vi "Change Default Font.vi"(0 "PDF Report IN":refnum<class "PDF Report Class.lvclass">, 2 "Font":T1={"Name"="Helvetica", "Size"=12.0, "Color"=0, "Style"={"Bold"=FALSE, "Italic"=FALSE, "Underline"=FALSE, "Strikeout"=FALSE}, "Type"={"Type&direction"=enum."Select", "Embedded"=FALSE, "Encoding"=""}}, 11 "error in (no error)":errorcluster) -> (4 "PDF Report OUT":refnum<class "PDF Report Class.lvclass">, 15 "error out":errorcluster)   [LabVIEW 2019, in "Exaprom PDF.lvlib" / "Font Class.lvclass"]
doc: "Set the default font of the PDF report.\n\n<B>FRANÇAIS</B>\nChange la police de caractères par défaut du rapport PDF.\n\nDeveloped by Jean-Marc Simard\nCopyright © 2010, Exaprom Inc.\nAll rights reserved.\nLicense: BSD\n\nWith iTextSharp 4.1.6 (http://itextsharp.sourceforge.net)\nunder Mozilla Public License Version 1.1\n(http://www.mozilla.org/MPL/MPL-1.1.html)"
uses:
  Font Class.lvclass
  PDF Report Class/PDF Report Class.lvclass
  Controls/Font Controls/Font complete cluster.ctl
  Controls/Font Controls/Font size.ctl
  Controls/Font Controls/Font color.ctl
  Controls/Font Controls/Type and encoding.ctl
  Controls/Text Controls/Unicode/Type and run direction.ctl
  Font Class.lvclass/Font Class.ctl
  Exaprom PDF.lvlib
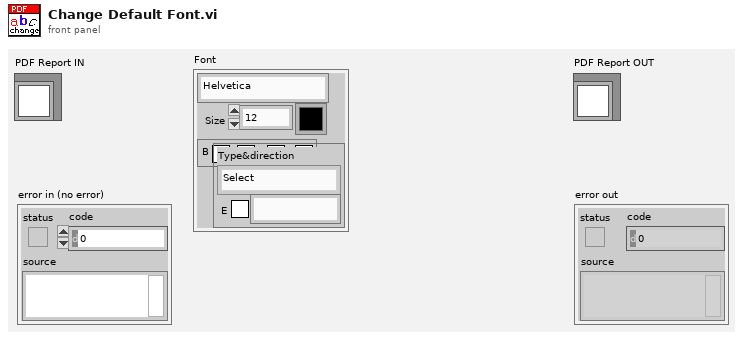
[diagram p1: front panel]
types:
  T1 = typedef "Exaprom PDF.lvlib/Font complete cluster.ctl" = cluster{"Name":string, "Size":T2, "Color":T3, "Style":cluster{"Bold":bool, "Italic":bool, "Underline":bool, "Strikeout":bool}, "Type":T4}
  T2 = typedef "Exaprom PDF.lvlib/Font size.ctl" = sgl
  T3 = typedef "Exaprom PDF.lvlib/Font color.ctl" = u32
  T4 = typedef "Exaprom PDF.lvlib/Type and encoding.ctl" = cluster{"Type&direction":T5, "Embedded":bool, "Encoding":string}
  T5 = typedef "Exaprom PDF.lvlib/Type and run direction.ctl" = enum16{"Select", "ASCII", "UTF-16", "UTF-16 (default)", "UTF-16 (LTR)", "UTF-16 (RTL)"}
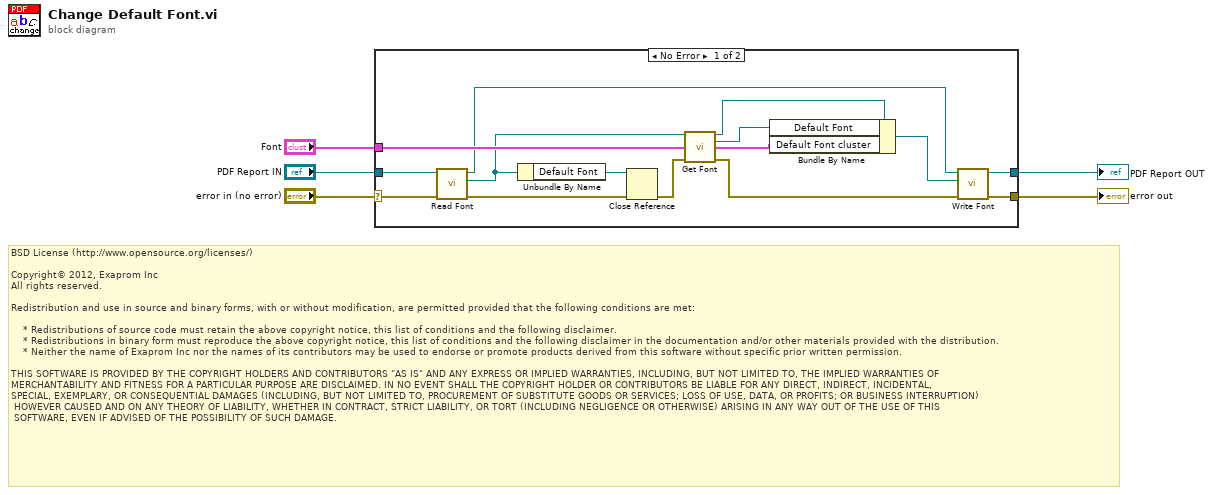
[diagram p0: block diagram]
diagram:
  # "BSD License (http://www.opensource.org/licenses/)\n\nCopyright© 2012, Exaprom Inc\nAll rights reserved.\n\nRedistribution and use in source and binary forms, with or without modification, are permitted provided that the following conditions are met:\n\n    * Redistributions of source code must retain the above copyright notice, this list of conditions and the following disclaimer.\n    * Redistributions in binary form must reproduce the above copyright notice, this list of conditions and the following disclaimer in the documentation and/or other materials provided with the distribution.\n    * Neither the name of Exaprom Inc nor the names of its contributors may be used to endorse or promote products derived from this software without specific prior written permission.\n\nTHIS SOFTWARE IS PROVIDED BY THE COPYRIGHT HOLDERS AND CONTRIBUTORS \"AS IS\" AND ANY EXPRESS OR IMPLIED WARRANTIES, INCLUDING, BUT NOT LIMITED TO, THE IMPLIED WARRANTIES OF \nMERCHANTABILITY AND FITNESS FOR A PARTICULAR PURPOSE ARE DISCLAIMED. IN NO EVENT SHALL THE COPYRIGHT HOLDER OR CONTRIBUTORS BE LIABLE FOR ANY DIRECT, INDIRECT, INCIDENTAL,\nSPECIAL, EXEMPLARY, OR CONSEQUENTIAL DAMAGES (INCLUDING, BUT NOT LIMITED TO, PROCUREMENT OF SUBSTITUTE GOODS OR SERVICES; LOSS OF USE, DATA, OR PROFITS; OR BUSINESS INTERRUPTION)\n HOWEVER CAUSED AND ON ANY THEORY OF LIABILITY, WHETHER IN CONTRACT, STRICT LIABILITY, OR TORT (INCLUDING NEGLIGENCE OR OTHERWISE) ARISING IN ANY WAY OUT OF THE USE OF THIS\n SOFTWARE, EVEN IF ADVISED OF THE POSSIBILITY OF SUCH DAMAGE."
  n1 = case shown="No Error" "error in (no error)" {
    selector: "error in (no error)" -> [w14 w22]
    tunnel: "PDF Report IN" -> [w13 w21]
    tunnel: [w7 w21] -> w4
    tunnel: "Font" -> [w19 _]
    tunnel: [w10 w22] -> w2
    frame No Error {
      n2 = call-dynamic "Read Font.vi"("error in (no error)"=w14, "PDF Report Class in"=w13) -> ("error out"=w15:errorcluster, "Font Class.lvclass"=w11:refnum<class "Font Class.lvclass">, "PDF Report Class out"=w8:refnum<class "PDF Report Class.lvclass">)  [unwired: 7 in]
      n3 = Unbundle By Name(w11) -> ("Default Font"=w12:refnum<k24>)
      n4 = Close Reference(reference=w12, error in (no error)=w15) -> (error out=w18:errorcluster)
      n5 = call "Get Font.vi"("Font"=w11, "Font IN"=w19, "error in (no error)"=w18) -> ("Font duplicate"=w17:refnum<class "Font Class.lvclass">, "Font"=w6:refnum<k24>, "Font OUT"=w16:T1, "error out"=w20:errorcluster)  [unwired: 8 in, 1 out]
      n6 = Bundle By Name(cluster=w17, "Default Font"=w6, "Default Font cluster"=w16) -> (w9:refnum<class "Font Class.lvclass">)
      n7 = call-dynamic "Write Font.vi"("error in (no error)"=w20, "Font Class.lvclass"=w9, "PDF Report Class in"=w8) -> ("error out"=w10:errorcluster, "PDF Report Class out"=w7:refnum<class "PDF Report Class.lvclass">)  [unwired: 7 in]
    }
    frame Error {
    }
  }
  "error out" <- w2
  "PDF Report OUT" <- w4
